vi "Level.vi"() -> ()   [LabVIEW 2011]
uses:
  Global.vi
panel:
  out "Waveform Chart":dbl(graph)
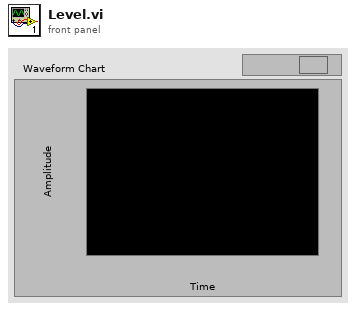
[diagram p1: front panel]
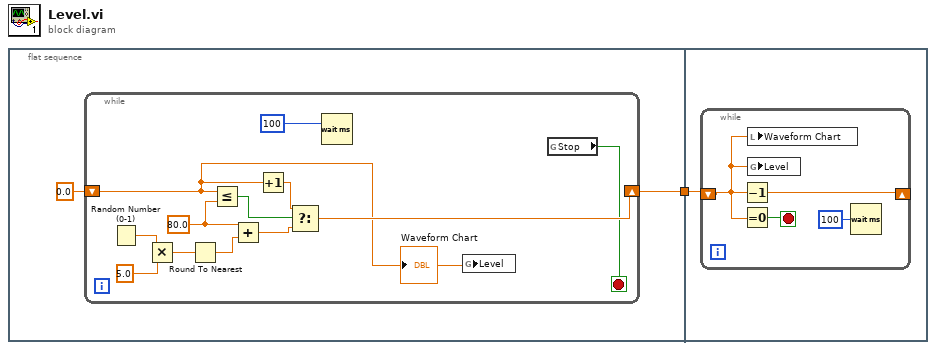
[diagram p0: block diagram]
diagram:
  n1 = flat-sequence {
    tunnel: [w2] -> w1
    tunnel: w1 -> [w16]
    frame #0 {
      n2 = while {
        shift-right: [w8] -> w2
        shift-left: 0.0 -> [w5]
        stop <- w4 stop-if-true
        w11 = 80.0
        n3 = Random Number (0-1)() -> (number: 0 to 1=w9:dbl)
        n4 = Multiply(x=w9, y=5.0) -> (x*y=w15:dbl)
        n5 = Round To Nearest(number=w15) -> (nearest integer value=w14:dbl)
        n6 = Less Or Equal?(x=w5, y=w11) -> (x <= y?=w7:bool)
        n7 = Add(x=w11, y=w14) -> (x+y=w13:dbl)
        n8 = Increment(x=w5) -> (x+1=w12:dbl)
        n9 = Select(t=w12, s=w7, f=w13) -> (s? t:f=w8:dbl)
        n10 = Wait (ms)(milliseconds to wait=100) -> ()  [unwired: 1 out]
        n11 = global write "Global.vi" "Level"(w5) -> ()
        n12 = global read "Global.vi" "Stop"() -> (w4:bool)
        "Waveform Chart" <- w5
      }
    }
    frame #1 {
      n13 = while {
        shift-right: [w18] -> _
        shift-left: w16 -> [w17]
        stop <- w20 stop-if-true
        n14 = Decrement(x=w17) -> (x-1=w18:dbl)
        n15 = Equal To 0?(x=w17) -> (x = 0?=w20:bool)
        n16 = local write "Waveform Chart"(w17) -> ()
        n17 = global write "Global.vi" "Level"(w17) -> ()
        n18 = Wait (ms)(milliseconds to wait=100) -> ()  [unwired: 1 out]
      }
    }
  }
